vi "Create Module UI Table.vi"(8 "error in (no error)":errorcluster, 10 "module datasets":T2[](array[typedef]), 11 "Color Names & Values":T1) -> (0 "error out":errorcluster, 2 "Array":T3[](array[typedef]), 3 "Color Names & Values 2":T1)   [LabVIEW 2015, in "GraphViz Mapping Visualizer.lvlib"]
doc: "Create Module Table from found Modules with default settings."
uses:
  GraphViz Mapping Visualizer.lvlib
  Sort Options.ctl
  Module Options.ctl
  <vilib>/NI/Tag Bus Module Framework/channel/TBM channel.lvclass
  <vilib>/NI/DCAF/Tag Editor Core/Configuration Editor/Classes/Engine Mappings/module information.ctl
  <vilib>/NI/DCAF/Tag Editor Core/Configuration Editor/Classes/Engine Mappings/Engine Mappings.lvclass
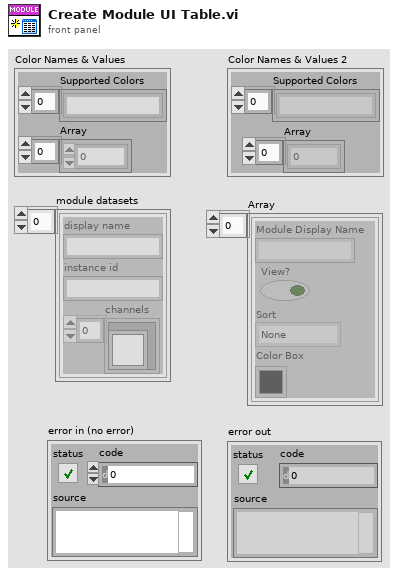
[diagram p1: front panel]
types:
  T1 = cluster{"Supported Colors":string[], "Array":u32[]}
  T2 = typedef "PL Framework Configuration Tool.lvlib/Engine Mappings.lvclass/module information.ctl" = cluster{"display name":string, "instance id":string, "channels":refnum<class "TBM channel.lvclass">[]}
  T3 = typedef "GraphViz Mapping Visualizer.lvlib/Module Options.ctl" = cluster{"Module Display Name":string, "View?":bool, "Sort":T4, "Color Box":u32}
  T4 = typedef "GraphViz Mapping Visualizer.lvlib/Sort Options.ctl" = enum16{"None", "All Ascending", "All Descending", "Channel Type Ascending", "Channel Type Descending"}
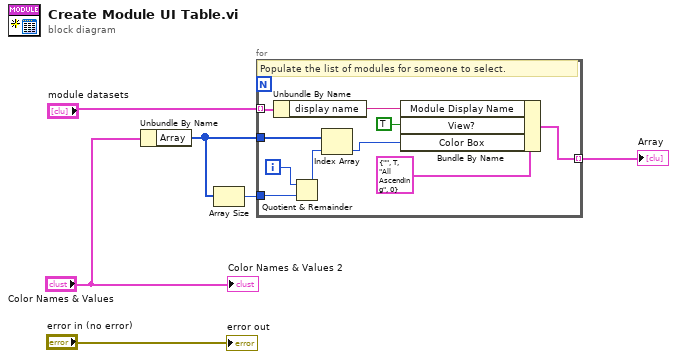
[diagram p0: block diagram]
diagram:
  n1 = Unbundle By Name("Color Names & Values") -> ("Array"=w4:u32[])
  n2 = Array Size(array=w4) -> (size(s)=w5:i32)
  n3 = for {
    tunnel: "module datasets" -> [w16] mode=indexing
    tunnel: [w12] -> w3 mode=indexing
    tunnel: w4 -> [w8]
    tunnel: w5 -> [w7]
    i -> [w10]
    # "Populate the list of modules for someone to select."
    n4 = Unbundle By Name(w16) -> ("display name"=w13:string)
    n5 = Quotient & Remainder(x=w10, y=w7) -> (x-y*floor(x/y)=w9:i32)  [unwired: 1 out]
    n6 = Index Array(array=w8, index=w9) -> (element=w11:u32)
    n7 = Bundle By Name(cluster=T3 {"Module Display Name"="", "View?"=TRUE, "Sort"=enum."All Ascending", "Color Box"=0} ("Cluster"), "Module Display Name"=w13, "View?"=TRUE, "Color Box"=w11) -> (w12:T3)
  }
  "Array" <- w3
  "error out" <- "error in (no error)"
  "Color Names & Values 2" <- "Color Names & Values"
